vi "Command to Bitwise Command.vi"(2 "OOB Command":u8) -> (4 "bit command":u64)   [LabVIEW 2021, in "CIFOutOfBand.lvclass"]
uses:
  CIFOutOfBand.lvclass
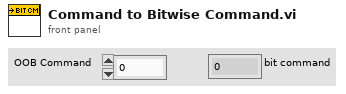
[diagram p1: front panel]
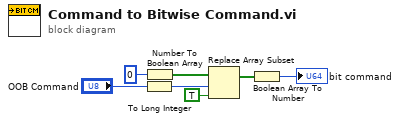
[diagram p0: block diagram]
diagram:
  n1 = To Long Integer(number="OOB Command") -> (32bit integer=w1:i32)
  n2 = Number To Boolean Array(number=u64 0) -> (Boolean array=w5:bool[])
  n3 = Replace Array Subset(array=w5, new element=TRUE ("new element/subarray"), index=w1) -> (w3:bool[])
  n4 = Boolean Array To Number(Boolean array=w3) -> (number=→"bit command":u64)
